vi "SPI Set Clock Frequency.vi"(8 "Error In":errorcluster, 9 "Target Clock Frequency":u32, 10 "SPI Channel":u8, 11 "LINX Device Config":T1) -> (0 "Error Out":errorcluster, 2 "Actual Frequency":u32, 3 "LINX Device Config":T1)   [LabVIEW 2019, in "LMH-LINX.lvlib" / "Device.lvlib"]
doc: "Set the bit order of the specified SPI Channel."
uses:
  <vilib>/MakerHub/LINX/Private/Device/Device.lvlib
  <vilib>/MakerHub/LINX/Private/Device/Type Defs/LINX Device Config.ctl
  <vilib>/MakerHub/LINX/Private/Type Defs/Interface.ctl
  <vilib>/MakerHub/LINX/Private/Device/Type Defs/TCP Config.ctl
  <vilib>/MakerHub/LINX/Private/Device/Type Defs/Channels.ctl
  <vilib>/MakerHub/LINX/Private/Type Defs/Error Type.ctl
  <vilib>/MakerHub/LINX/LMH-LINX.lvlib
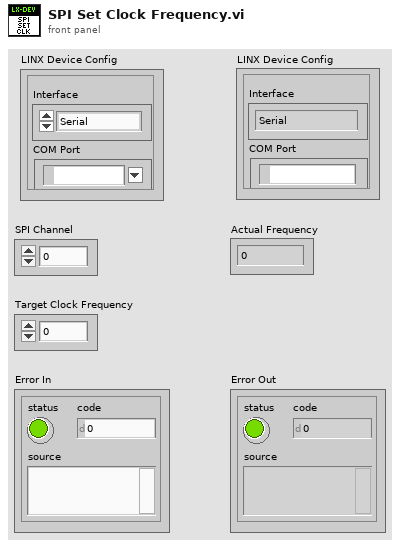
[diagram p1: front panel]
types:
  T1 = typedef "LMH-LINX.lvlib/Device.lvlib/LINX Device Config.ctl" = cluster{"Interface":T2, "COM Port":refnum<visa-resource-name>, "TCP Configuration":T3, "Device Family":u8, "Device ID":u8, "Device Name":string, "TCP Ref":refnum<k5>, "Channels":T4}
  T2 = typedef "LMH-LINX.lvlib/Interface.ctl" = enum16{"Serial", "TCP"}
  T3 = typedef "LMH-LINX.lvlib/Device.lvlib/TCP Config.ctl" = cluster{"IP Address":string, "Port":u16}
  T4 = typedef "LMH-LINX.lvlib/Channels.ctl" = cluster{"DI":u8[], "DO":u8[], "AI":u8[], "AO":u8[], "PWM":u8[], "QE":u8[], "UART":u8[], "I2C 2":u8[], "SPI":u8[], "CAN":u8[], "Servo":u8[], "AI Ref (V)":dbl, "AI Resolution (Bits)":u8, "AO Ref (V)":dbl, "AO Resolution (Bits)":u8}
  T5 = typedef "LMH-LINX.lvlib/Error Type.ctl" = enum16{"Unknown", "Timeout", "Corrupt Return Packet", "Unable To Connect", "Command Not Supported", "Channel DNE", "Invalid COM Config", "Firmware Version Mismatch", "myRIO Support", "CMD Specific Error", "Local IO Not Supported"}
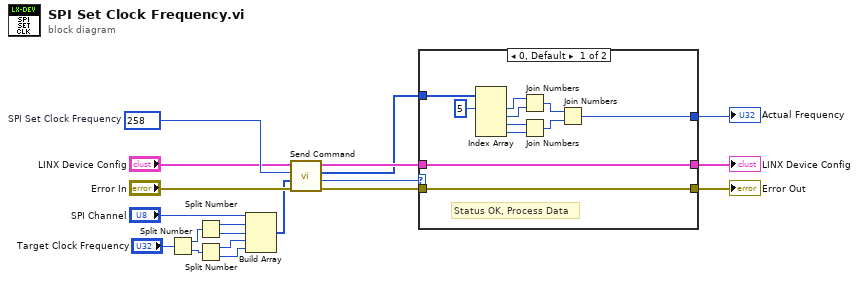
[diagram p0: block diagram]
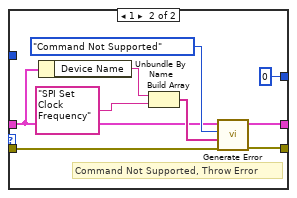
[diagram p2: hidden frame]
diagram:
  w18 = u16 258  # SPI Set Clock Frequency
  n1 = Split Number(x="Target Clock Frequency") -> (hi(x)=w8:u16, lo(x)=w9:u16)
  n2 = Split Number(x=w8) -> (hi(x)=w7:u8, lo(x)=w6:u8)
  n3 = Split Number(x=w9) -> (hi(x)=w5:u8, lo(x)=w4:u8)
  n4 = Build Array("SPI Channel", w7, w6, w5, w4) -> (w11:u8[])
  n5 = call <vilib>:"Send Command.vi"("Error In"="Error In", "ARGS"=w11, "CMD"=w18, "LINX Device Config"="LINX Device Config") -> ("Error Out"=w13:errorcluster, "Status"=w3:u8, "Response"=w2:u8[], "LINX Device Config"=w15:T1)  [unwired: 4 in]
  n6 = case shown="0, Default" w3 {
    tunnel: [w30 w37] -> w16
    tunnel: w15 -> [w30 w33]
    tunnel: [w29 w38] -> w14
    tunnel: w13 -> [w29 w39]
    tunnel: w2 -> [w28 _]
    tunnel: [w20 u32 0] -> w1
    frame 0, Default {
      # "Status OK, Process Data"
      n7 = Index Array(array=w28, index #1=5 ("index")) -> (element #1=w26:u8, element #2=w25:u8, element #3=w24:u8, element #4=w23:u8)  [unwired: 3 in]
      n8 = Join Numbers(hi=w26, lo=w25) -> ((hi.lo)=w22:u16)
      n9 = Join Numbers(hi=w24, lo=w23) -> ((hi.lo)=w21:u16)
      n10 = Join Numbers(hi=w22, lo=w21) -> ((hi.lo)=w20:u32)
    }
    frame 1 {
      # "Command Not Supported, Throw Error"
      n11 = Unbundle By Name(w33) -> ("Device Name"=w32:string)
      n12 = Build Array(w32, "SPI Set Clock Frequency") -> (w34:string[])
      n13 = call <vilib>:"Generate Error.vi"("Error In"=w39, "Arguments"=w34, "Error Type"=Error_Type."Command Not Supported", "LINX Device Config"=w33) -> ("Error Out"=w38:errorcluster, "Dup LINX Device Config"=w37:T1)  [unwired: 6 in]
    }
  }
  "Error Out" <- w14
  "LINX Device Config" <- w16
  "Actual Frequency" <- w1
